vi "Stitch two images.vi"(0 "Timelapse Image in":T2, 1 "Which tier?":enum16{"Top tier", "Bottom tier"}(ring), 3 "Name for resampled Image 1":string="First", 5 "Ctrl refs":T1, 9 "Gobal frame number in Timelapse data/master video (1 based)":i32, 11 "error in (no error)":errorcluster, 12 "Initial frame":bool, 13 "Output X Resolution":i32=500, 14 "Name for resampled Image 2":string="Second") -> (4 "Bottom tier Stitched Image":T2(plugin-control), 15 "error out":errorcluster)   [LabVIEW 2020]
uses:
  <vilib>/vision/Image Controls.llb/IMAQ Image.ctl
  Typedefs/8-bit video export window ctrl refs.ctl
  Patch-Vol video generator/Typedefs/Bright-Contr-Gamma cluster.ctl
  Typedefs/Speed graph behaviour enum.ctl
  Functional Imaging Viewer/Typedefs/Get-Set-Clear Control.ctl
  Typedefs/Image stitching positions.ctl
  <vilib>/vision/NI_Vision_Development_Module.lvlib
panel:
  in  "AVI File Path":path=path "F:/Recovered data 03-24-2015 at 11_16_03/NTFS 1/LostFiles1/TimeLapse 03_10_2014 17-26-28 zoom1_50ns_MF_export/Green Channel 1.avi"
  out "Timelapse image":T2(plugin-control)
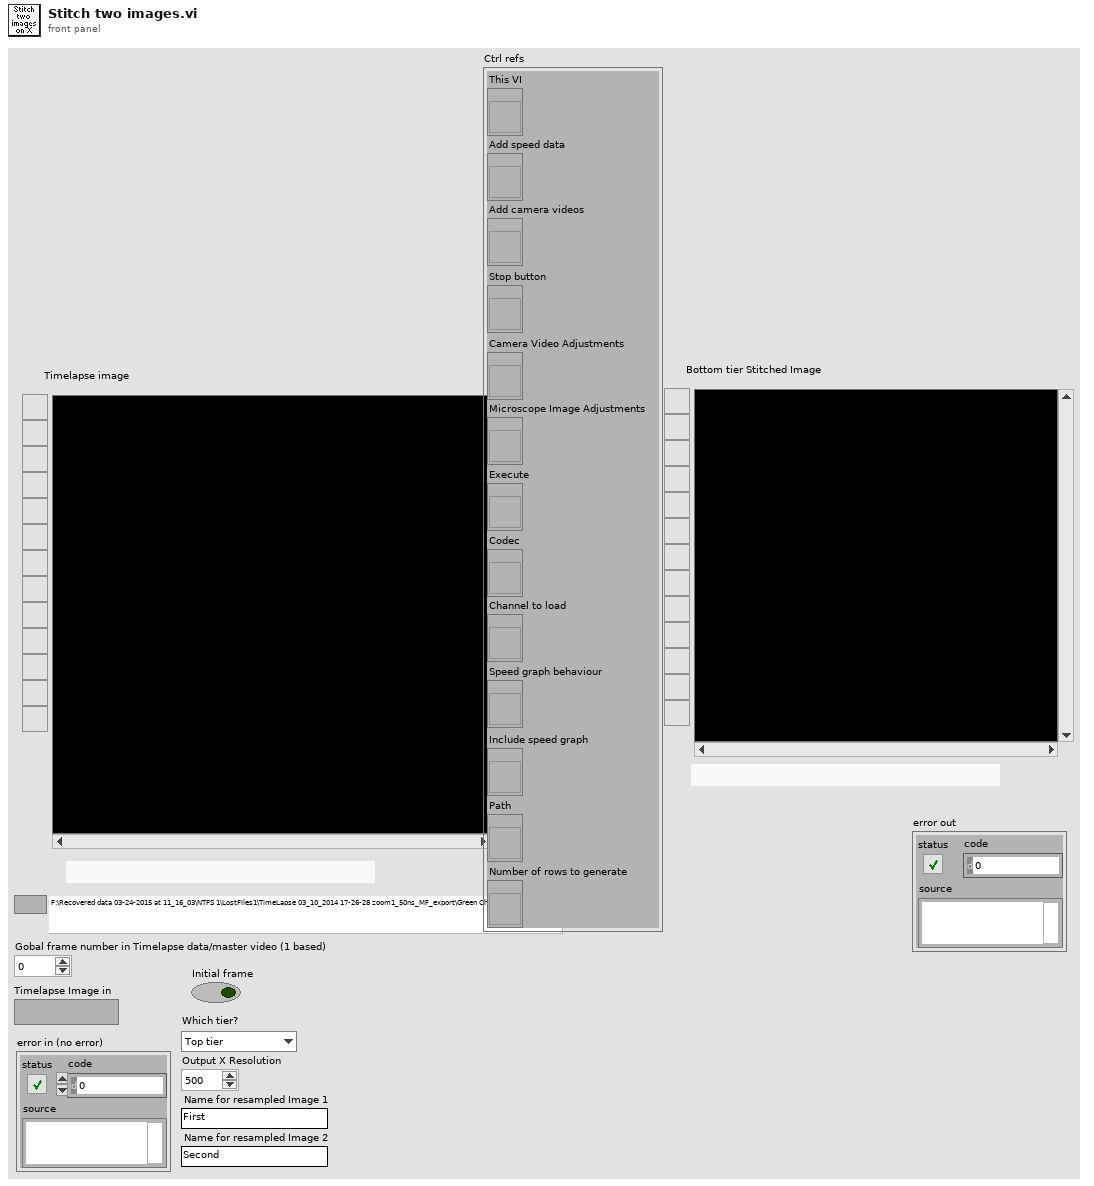
[diagram p1: front panel]
types:
  T1 = typedef "8-bit video export window ctrl refs.ctl" = cluster{"This VI":refnum<vi>, "Add speed data":refnum<vi>, "Add camera videos":refnum<vi>, "Stop button":refnum<vi>, "Camera Video Adjustments":refnum<vi>, "Microscope Image Adjustments":refnum<vi>, "Execute":refnum<vi>, "Codec":refnum<vi>, "Channel to load":refnum<vi>, "Speed graph behaviour":refnum<vi>, "Include speed graph":refnum<vi>, "Number of rows to generate":refnum<vi>, "Path":refnum<vi>}
  T2 = typedef "IMAQ Image.ctl" = refnum<image>
  T3 = typedef "Get-Set-Clear Control.ctl" = enum16{"Get", "Set", "Clear"}
  T4 = typedef "Image stitching positions.ctl" = enum16{"Top left", "Top right", "Bottom left", "Bottom right", "Not used"}
  T5 = cluster{"Image 1 position":T4, "Image 2 position":T4}
  T6 = typedef "Image Type" = u32
  T7 = typedef "IMAQ AVI2 Refnum.ctl" = refnum<k20>
  T8 = typedef "Cam videos cluster.ctl" = cluster{"Vid 1":T2, "Vid 2":T2, "Vid 3":T2, "Vid 4":T2, "Vid1 Rel time (ms)":u32, "Vid2 Rel time (ms)":u32, "Vid3 Rel time (ms)":u32, "Vid4 Rel time (ms)":u32}
  T9 = typedef "Stitch layout spec cluster.ctl" = cluster{"Timelapse image":cluster{"Image position":T4}, "Cam 1":cluster{"Image position":T4}, "Cam 2":cluster{"Image position":T4}, "Cam 3":cluster{"Image position":T4}, "Cam 4":cluster{"Image position":T4}}
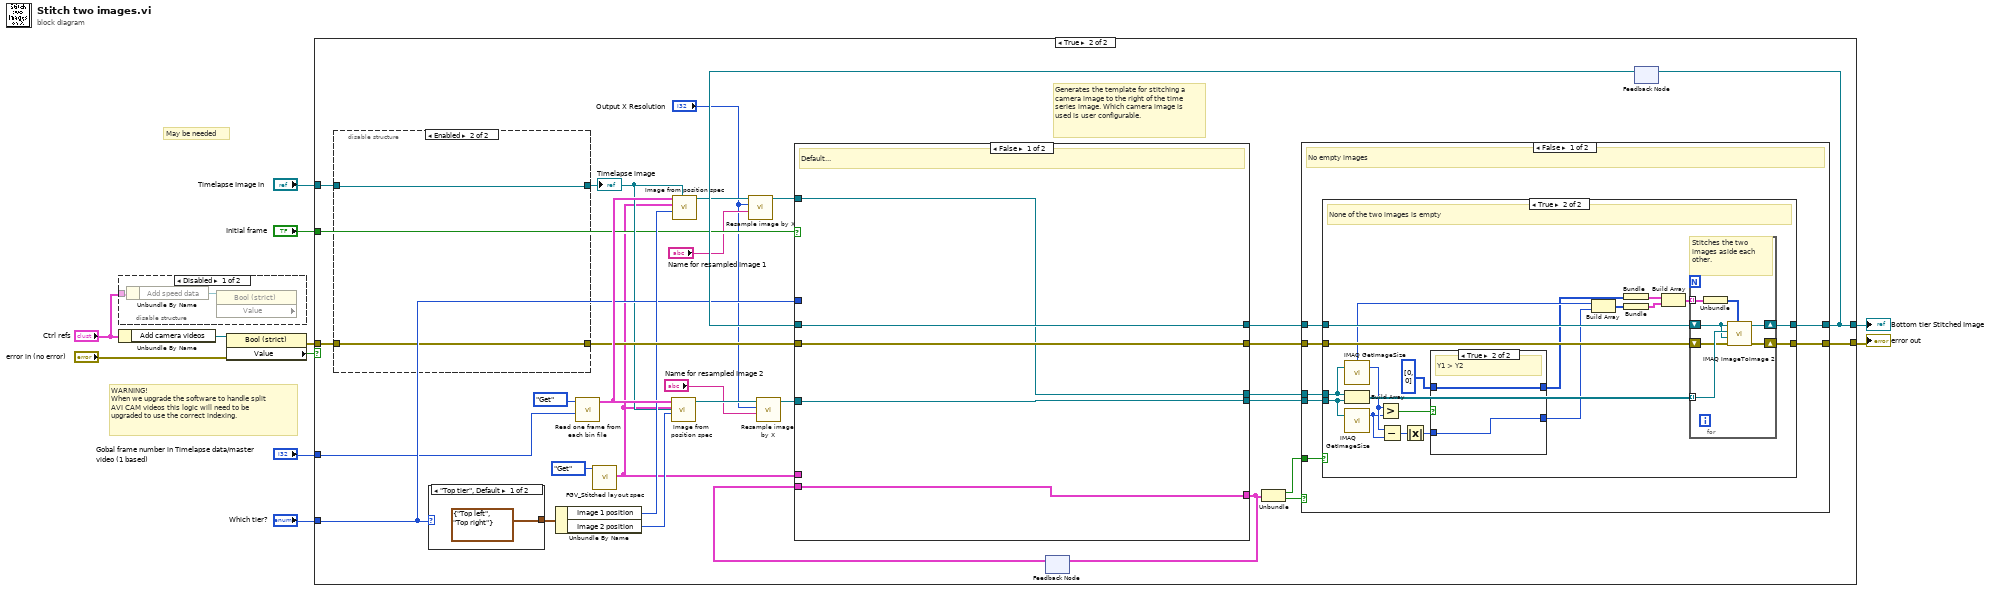
[diagram p0: block diagram]
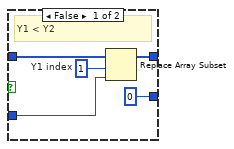
[diagram p5: hidden frame]
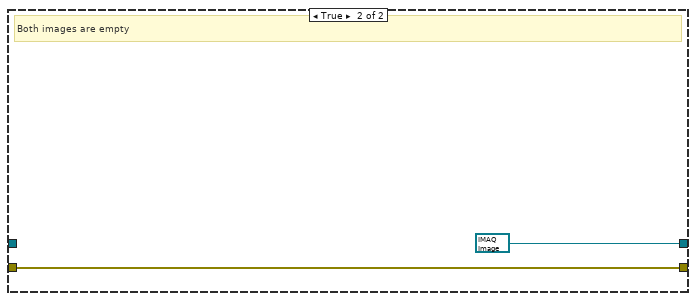
[diagram p6: hidden frame]
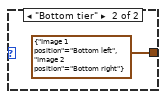
[diagram p7: hidden frame]
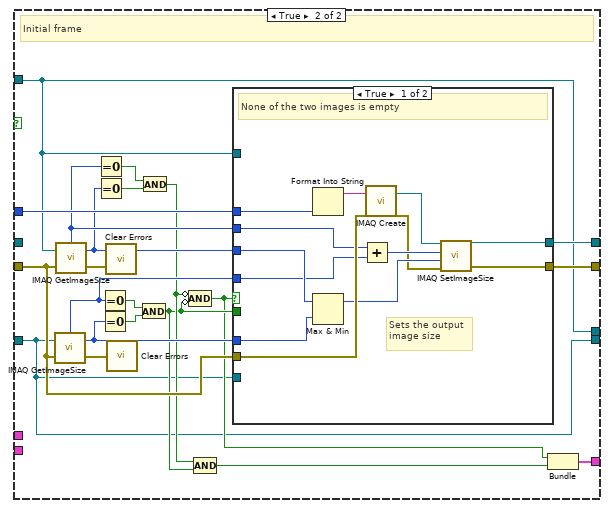
[diagram p8: hidden frame]
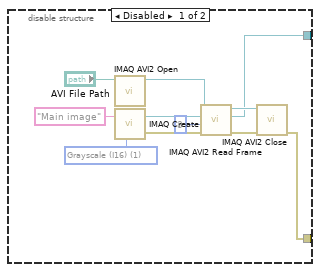
[diagram p11: hidden frame]
diagram:
  # "WARNING!\nWhen we upgrade the software to handle split AVI CAM videos this logic will need to be upgraded to use the correct indexing."
  # "May be needed"
  n1 = disable-structure shown="Disabled" {
    disable-tunnel: "Ctrl refs" -> [w12 _]
    frame Disabled {
      n2 = Unbundle By Name(w12) -> ("Add speed data"=w13:refnum<vi>)
      n3 = property class="Bool (strict)" props=["Value"](reference=w13) -> ()  [unwired: 1 in, 3 out]
    }
    frame Enabled {
    }
  }
  n4 = Unbundle By Name("Ctrl refs") -> ("Add camera videos"=w9:refnum<vi>)
  n5 = property class="Bool (strict)"(reference=w9, error in="error in (no error)") -> (error out=w6:errorcluster, "Value"=w8:bool)  [unwired: 1 out]
  n6 = case shown="True" w8 {
    tunnel: [w15 w39] -> w11
    tunnel: [w14 w40] -> w10
    tunnel: "Timelapse Image in" -> [w15 w47]
    tunnel: w6 -> [w14 w46]
    tunnel: "Initial frame" -> [_ w29]
    tunnel: "Gobal frame number in Timelapse data/master video (1 based)" -> [_ w16]
    tunnel: "Which tier?" -> [_ w32]
    frame False {
    }
    frame True {
      # "Generates the template for stitching a camera image to the right of the time series image. Which camera image is used is user configurable."
      n7 = disable-structure shown="Enabled" {
        disable-tunnel: [w150 w161] -> w30
        disable-tunnel: [w149 w160] -> w36
        disable-tunnel: w47 -> [_ w161]
        disable-tunnel: w46 -> [_ w160]
        frame Disabled {
          w157 = T6 1 items=["Grayscale (U8)", "Grayscale (I16)", "Grayscale (SGL)", "Complex (CSG)", "RGB (U32)", "HSL (U32)", "RGB (U64)", "Grayscale (U16)"] ("Image Type")
          n8 = call "IMAQ AVI2 Open"("AVI File Path"="AVI File Path") -> ("AVI Refnum"=w159:T7)  [unwired: 9 in, 1 out]
          n9 = call "IMAQ Create"("Image Name"="Main image", "Image Type"=w157) -> ("New Image"=w155:T2, "error out"=w154:errorcluster)  [unwired: 3 in]
          n10 = call "IMAQ AVI2 Read Frame"("error in (no error)"=w154, "Frame Number"=u32 3, "Image"=w155, "AVI Refnum"=w159) -> ("error out"=w153:errorcluster, "Image Out"=w150:T2, "AVI Refnum (duplicate)"=w158:T7)  [unwired: 5 in]
          n11 = call "IMAQ AVI2 Close"("error in (no error)"=w153, "AVI Refnum"=w158) -> ("error out"=w149:errorcluster)  [unwired: 9 in]
        }
        frame Enabled {
        }
      }
      "Timelapse image" <- w30
      n12 = case shown="\"Top tier\", Default" w32 {
        tunnel: [T5 {"Image 1 position"=enum."Top left", "Image 2 position"=enum."Top right"} ("Top tier") T5 {"Image 1 position"=enum."Bottom left", "Image 2 position"=enum."Bottom right"} ("Bottom tier")] -> w35
        frame "Top tier", Default {
        }
        frame "Bottom tier" {
        }
      }
      n13 = Unbundle By Name(w35) -> ("Image 1 position"=w34:T4, "Image 2 position"=w33:T4)
      n14 = call "Read one frame from each bin file.vi"("Master video's frame number (unity-based)"=w16, "Get/set"=Get-Set-Clear_Control."Get" ("GEt set .bin refs")) -> ("Cam videos cluster"=w37:T8)  [unwired: 8 in, 1 out]
      n15 = call "FGV_Stitched layout spec.vi"("Function"=Get-Set-Clear_Control."Get") -> ("Stitch layout spec"=w24:T9)  [unwired: 9 in, 1 out]
      n16 = call "Image from position spec.vi"("Timelapse image"=w30, "Image position"=w33, "Stitch layout spec"=w24, "Cam videos cluster"=w37) -> ("Selected image"=w21:T2)  [unwired: 7 in]
      n17 = call "Image from position spec.vi"("Timelapse image"=w30, "Image position"=w34, "Stitch layout spec"=w24, "Cam videos cluster"=w37) -> ("Selected image"=w22:T2)  [unwired: 7 in]
      n18 = call "Resample image by X.vi"("Resampled Image Name"="Name for resampled Image 1", "X Resolution"="Output X Resolution", "Refnum in"=w22) -> ("Refnum out"=w23:T2)  [unwired: 8 in]
      n19 = call "Resample image by X.vi"("Resampled Image Name"="Name for resampled Image 2", "X Resolution"="Output X Resolution", "Refnum in"=w21) -> ("Refnum out"=w20:T2)  [unwired: 8 in]
      n20 = feedback #1() -> (w31:cluster{bool, bool})  [unwired: 1 in]
      n21 = feedback #2() -> (w38:T2)  [unwired: 1 in]
      n22 = case shown="False" w29 {
        tunnel: w36 -> [w99 w109]
        tunnel: [w99 w119] -> w44
        tunnel: [w98 w120] -> w43
        tunnel: [w97 w101] -> w42
        tunnel: [w96 w100] -> w41
        tunnel: w38 -> [w98 _]
        tunnel: w24 -> [_ _]
        tunnel: w20 -> [w96 w100]
        tunnel: w23 -> [w97 w101]
        tunnel: w32 -> [_ w118]
        tunnel: w31 -> [w95 _]
        tunnel: [w95 w102] -> w28
        frame False {
          # "Default..."
        }
        frame True {
          # "Initial frame"
          n23 = call "IMAQ GetImageSize"("Image"=w100, "error in (no error)"=w109) -> ("Y Resolution"=w111:i32, "X Resolution"=w110:i32, "error out"=w108:errorcluster)  [unwired: 2 in]
          n24 = call "IMAQ GetImageSize"("Image"=w101, "error in (no error)"=w109) -> ("Y Resolution"=w116:i32, "X Resolution"=w117:i32, "error out"=w107:errorcluster)  [unwired: 2 in]
          n25 = Equal To 0?(x=w117) -> (x = 0?=w115:bool)
          n26 = Equal To 0?(x=w116) -> (x = 0?=w114:bool)
          n27 = Equal To 0?(x=w110) -> (x = 0?=w113:bool)
          n28 = Equal To 0?(x=w111) -> (x = 0?=w112:bool)
          n29 = call <vilib>:"Clear Errors.vi"("error in (no error)"=w107) -> ()  [unwired: 5 in, 2 out]
          n30 = call <vilib>:"Clear Errors.vi"("error in (no error)"=w108) -> ()  [unwired: 5 in, 2 out]
          n31 = And(x=w113, y=w112) -> (x .and. y?=w105:bool)
          n32 = And(x=w115, y=w114) -> (x .and. y?=w106:bool)
          n33 = Compound Arithmetic op=AND(invert w106, invert w105) -> (w104:bool)
          n34 = Compound Arithmetic op=AND(w106, w105) -> (w103:bool)
          n35 = case shown="True" w104 {
            tunnel: [w133 w144] -> w120
            tunnel: w109 -> [w132 w143]
            tunnel: [w131 w142] -> w119
            tunnel: w118 -> [w130 w141]
            tunnel: w117 -> [w129 w140]
            tunnel: w116 -> [w128 w139]
            tunnel: w111 -> [w127 w138]
            tunnel: w110 -> [w126 w137]
            tunnel: w105 -> [_ w136]
            tunnel: w101 -> [_ w135]
            tunnel: w100 -> [_ w134]
            frame True {
              # "Sets the output image size"
              # "None of the two images is empty"
              n36 = Format Into String(w130) -> (resulting string=w121:string)  [unwired: 3 in, 1 out]
              n37 = Max & Min(x=w128, y=w127) -> (max(x,y)=w124:i32)  [unwired: 1 out]
              n38 = Add(x=w129, y=w126) -> (x+y=w125:i32)
              n39 = call "IMAQ Create"("Image Name"=w121, "error in (no error)"=w132) -> ("New Image"=w123:T2, "error out"=w122:errorcluster)  [unwired: 2 in, 1 out]
              n40 = call "IMAQ SetImageSize"("error in (no error)"=w122, "Y Resolution"=w124, "X Resolution"=w125, "Image"=w123) -> ("error out"=w131:errorcluster, "Image Out"=w133:T2)  [unwired: 1 out]
            }
            frame False {
              # "One or both images are empty."
              n41 = case shown="False" w136 {
                tunnel: [w146 w147] -> w144
                tunnel: w143 -> [w145 w148]
                tunnel: [w145 w148] -> w142
                tunnel: w141 -> [_ _]
                tunnel: w140 -> [_ _]
                tunnel: w139 -> [_ _]
                tunnel: w138 -> [_ _]
                tunnel: w137 -> [_ _]
                tunnel: w135 -> [_ w147]
                tunnel: w134 -> [w146 _]
                frame False {
                }
                frame True {
                }
              }
            }
          }
          n42 = Bundle(w104, w103) -> (w102:cluster{bool, bool})  [unwired: 1 in]
        }
      }
      n43 = feedback-in #1(w28) -> ()
      n44 = Unbundle(w28) -> (w27:bool, w26:bool)
      n45 = case shown="False" w26 {
        tunnel: w44 -> [w54 w92]
        tunnel: w43 -> [w53 _]
        tunnel: w42 -> [w52 _]
        tunnel: w41 -> [w51 _]
        tunnel: [w50 w92] -> w40
        tunnel: [w49 T2 refnum ("Selected image")] -> w39
        tunnel: w27 -> [w48 _]
        frame False {
          # "No empty images"
          n46 = case shown="True" w48 {
            tunnel: w54 -> [w55 w76]
            tunnel: w53 -> [w56 w75]
            tunnel: w52 -> [_ w71]
            tunnel: w51 -> [_ w70]
            tunnel: [w55 w73] -> w50
            tunnel: [w56 w72] -> w49
            frame False {
              # "One of the images is empty"
            }
            frame True {
              # "None of the two images is empty"
              n47 = call "IMAQ GetImageSize"("Image"=w71) -> ("Y Resolution"=w67:i32, "X Resolution"=w62:i32)  [unwired: 1 in, 3 out]
              n48 = Build Array(w71, w70) -> (w74:T2[])
              n49 = call "IMAQ GetImageSize"("Image"=w70) -> ("Y Resolution"=w66:i32)  [unwired: 1 in, 4 out]
              n50 = Greater?(x=w67, y=w66) -> (0:w68:bool)
              n51 = Subtract(x=w67, y=w66) -> (x-y=w65:i32)
              n52 = Absolute Value(x=w65) -> (abs(x)=w64:i32)
              n53 = case shown="True" w68 {
                tunnel: i32[] [0, 0] -> [w80 w83]
                tunnel: [w79 w83] -> w59
                tunnel: w64 -> [w78 w82]
                tunnel: [0 ("new element/subarray") w82] -> w61
                frame False {
                  w81 = 1  # Y1 index
                  # "Y1 < Y2"
                  n54 = Replace Array Subset(array=w80, new element=w78, index=w81) -> (w79:i32[])
                }
                frame True {
                  # "Y1 > Y2"
                }
              }
              n55 = Build Array(w62, w61) -> (w60:i32[])
              n56 = Bundle(w59) -> (w57:cluster{i32[]})  [unwired: 1 in]
              n57 = Bundle(w60) -> (w58:cluster{i32[]})  [unwired: 1 in]
              n58 = Build Array(w57, w58) -> (w69:cluster{i32[]}[])
              n59 = for {
                tunnel: w74 -> [w90] mode=indexing
                shift-right: [w89] -> w72
                shift-left: w75 -> [w88]
                shift-right: [w87] -> w73
                shift-left: w76 -> [w86]
                tunnel: w69 -> [w85] mode=indexing
                # "Stitches the two images aside each other."
                n60 = Unbundle(w85) -> (w84:i32[])
                n61 = call "IMAQ ImageToImage 2"("Offset Left/Top"=w84, "error in (no error)"=w86, "Image Dst"=w88, "Image Src (Small)"=w90, "Image Src (Large)"=w88) -> ("error out"=w87:errorcluster, "Image Dst Out"=w89:T2)  [unwired: 1 in, 4 out]
              }
            }
          }
        }
        frame True {
          # "Both images are empty"
        }
      }
      n62 = feedback-in #2(w39) -> ()
    }
  }
  "Bottom tier Stitched Image" <- w11
  "error out" <- w10
